vi "add_dummy_feature.vi"(8 "error in":errorcluster caption="entrée d'erreur", 9 "X":string[][](array[string]), 10 "Type X":T1(ring), 11 "add_dummy_feature":cluster{"value":dbl}={"value"=1.0}) -> (0 "error out":errorcluster caption="sortie d'erreur", 3 "Data":T2)   [LabVIEW 2020]
doc: "Augment dataset with an additional dummy feature.\n\nThis is useful for fitting an intercept term with implementations which cannot otherwise fit it directly.\n\nParameters : \n\n- X : {array-like, sparse matrix}, shape [n_samples, n_features]\nData.\n\n- value : float\nValue to use for the dummy feature.\n\nReturns : \n\n- X : {array, sparse matrix}, shape [n_samples, n_features + 1]\nSame data with dummy feature added as first column."
uses:
  add_dummy_feature.lvclass
panel:
  out "add_dummy_feature.lvclass":refnum<class "add_dummy_feature.lvclass">
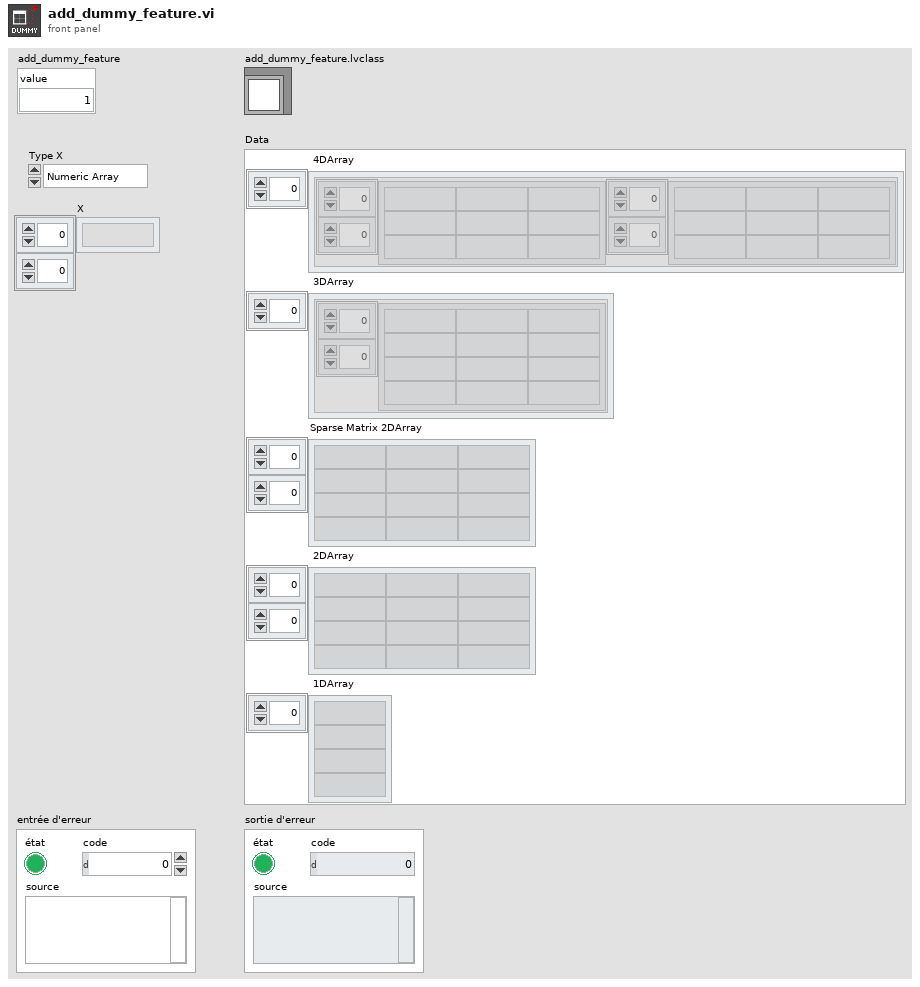
[diagram p1: front panel]
types:
  T1 = enum16{"Numeric Array", "String Array", "Sparse"}
  T2 = cluster{" 4DArray":cluster{"1":string[][], "2":string[][]}[], " 3DArray":cluster{"Tableau":string[][]}[], "Sparse Matrix 2DArray":string[][], " 2DArray":string[][], " 1DArray":string[]}
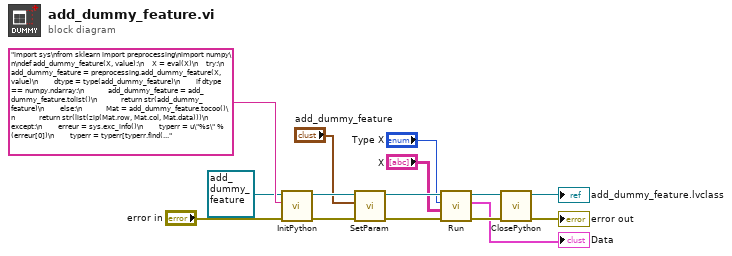
[diagram p0: block diagram]
diagram:
  n1 = call-dynamic "InitPython.vi"("error in (no error)"="error in", "Python Instruction"="import sys\nfrom sklearn import preprocessing\nimport numpy\n\ndef add_dummy_feature(X, value):\n    X = eval(X)\n    try:\n        add_dummy_feature = preprocessing.add_dummy_feature(X, value)\n        dtype = type(add_dummy_feature)\n        if dtype == numpy.ndarray:\n            add_dummy_feature = add_dummy_feature.tolist()\n            return str(add_dummy_feature)\n        else:\n            Mat = add_dummy_feature.tocoo()\n            return str(list(zip(Mat.row, Mat.col, Mat.data)))\n    except:\n        erreur = sys.exc_info()\n        typerr = u\"%s\" % (erreur[0])\n        typerr = typerr[typerr.find(\"'\")+1:typerr.rfind(\"'\")]\n        msgerr = u\"%s\" % (erreur[1])\n        message = str('/!\\\\ {0} : {1}'. format(typerr,msgerr))\n        return message ", "Scikit-learn en entrée"=refnum<class "add_dummy_feature.lvclass"> refnum ("add_dummy_feature.lvclass")) -> ("error out"=w10:errorcluster, "Scikit-learn en sortie"=w12:refnum<class "add_dummy_feature.lvclass">)  [unwired: 7 in]
  n2 = call-dynamic "SetParam.vi"("error in (no error)"=w10, "add_dummy_feature"="add_dummy_feature", "add_dummy_feature.lvclass"=w12) -> ("error out"=w8:errorcluster, "add_dummy_feature.lvclass"=w9:refnum<class "add_dummy_feature.lvclass">)  [unwired: 7 in]
  n3 = call-dynamic "Run.vi"("error in (no error)"=w8, "X"="X", "Type X"="Type X", "add_dummy_feature.lvclass"=w9) -> ("error out"=w5:errorcluster, "Data"=→"Data":T2, "add_dummy_feature.lvclass"=w6:refnum<class "add_dummy_feature.lvclass">)  [unwired: 5 in]
  n4 = call-dynamic "ClosePython.vi"("error in (no error)"=w5, "Scikit-learn en entrée"=w6) -> ("error out"=→"error out":errorcluster, "Scikit-learn en sortie"=→"add_dummy_feature.lvclass":refnum<class "add_dummy_feature.lvclass">)  [unwired: 8 in]
